vi "Configure List Band.vi"(5 "High Limit (0)":dbl, 7 "Low Limit (0)":dbl, 8 "error in (no error)":errorcluster, 9 "Limit Mode (0:Off)":u16(ring) items=["Off", "Primary", "Secondary"], 10 "Point No. (1)":i32=1, 11 "VISA resource name":refnum<visa-resource-name>) -> (0 "error out":errorcluster, 3 "VISA resource name out":refnum<visa-resource-name>)   [LabVIEW 2016, in "Agilent E4980.lvlib"]
doc: "Sets the limit values of the limit function for the list sweep measurement."
uses:
  <instrlib>/Agilent E4980/Agilent E4980.lvlib
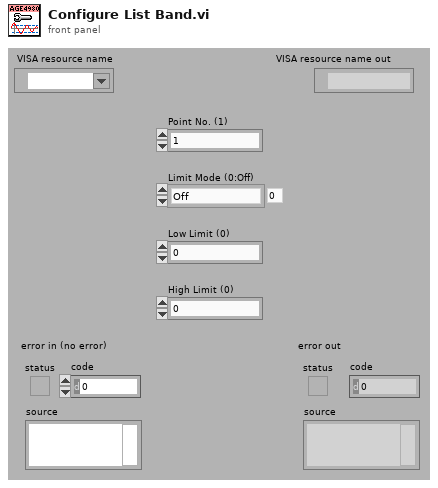
[diagram p1: front panel]
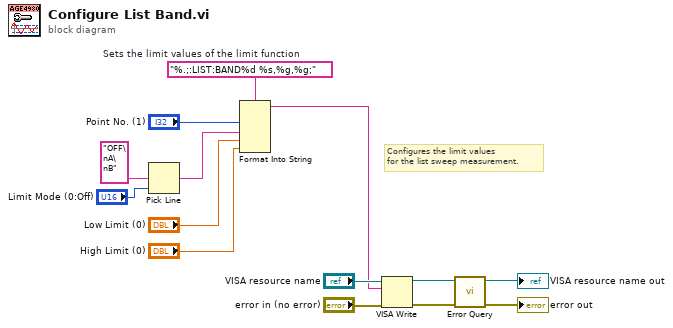
[diagram p0: block diagram]
diagram:
  w14 = "%.;:LIST:BAND%d %s,%g,%g;"  # Sets the limit values of the limit function
  # "Configures the limit values\nfor the list sweep measurement."
  n1 = Pick Line(multi-line string="OFF\nA\nB", line index="Limit Mode (0:Off)") -> (output string=w11:string)  [unwired: 1 in]
  n2 = Format Into String(format string=w14, "Point No. (1)", w11, "Low Limit (0)", "High Limit (0)") -> (resulting string=w6:string)  [unwired: 2 in, 1 out]
  n3 = VISA Write(VISA resource name="VISA resource name", write buffer=w6, error in (no error)="error in (no error)") -> (VISA resource name out=w5:refnum<visa-resource-name>, error out=w4:errorcluster)  [unwired: 1 out]
  n4 = call <instrlib>:"Error Query.vi"("error in (no error)"=w4, "VISA resource name"=w5) -> ("error out"=→"error out":errorcluster, "VISA resource name out"=→"VISA resource name out":refnum<visa-resource-name>)  [unwired: 6 in, 2 out]
